vi "LeftButtonUp.vi"(8 "Error in (no error)":errorcluster, 11 "Click?":bool=TRUE) -> (0 "Error out":errorcluster)   [LabVIEW 2013]
uses:
  user32.dll
  Linux VIs/guiLib.so
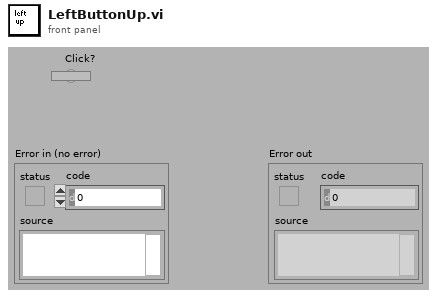
[diagram p1: front panel]
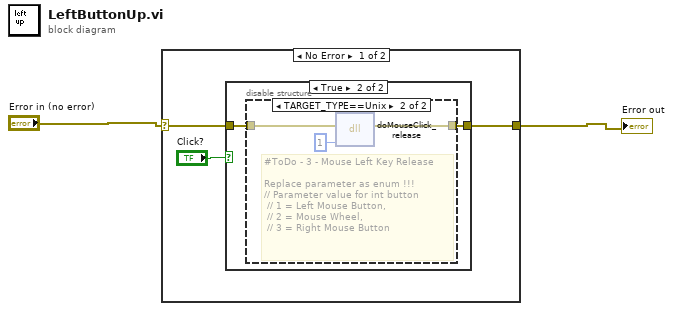
[diagram p0: block diagram]
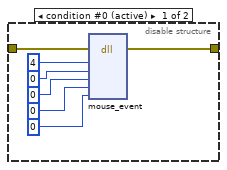
[diagram p3: hidden frame]
diagram:
  n1 = case shown="No Error" "Error in (no error)" {
    selector: "Error in (no error)" -> [w5 w19]
    tunnel: [w4 w19] -> w2
    frame No Error {
      n2 = case shown="True" "Click?" {
        tunnel: w5 -> [w6 w8]
        tunnel: [w6 w7] -> w4
        frame False {
        }
        frame True {
          n3 = disable-structure shown="TARGET_TYPE==Unix" {
            disable-tunnel: w8 -> [w10 w18]
            disable-tunnel: [w9 w17] -> w7
            frame condition #0 (active) {
              n4 = dll-call lib="user32.dll" fn="mouse_event"(error in=w10, "dwFlags"=u32 4, "dx"=u32 0, "dy"=u32 0, "dwData"=u32 0, "dxExtraInfo"=u32 0) -> (error out=w9:errorcluster)  [unwired: 7 in, 2 out]
            }
            frame condition #1 {
              # "#ToDo - 3 - Mouse Left Key Release\n\nReplace parameter as enum !!!\n// Parameter value for int button\n\t// 1 = Left Mouse Button, \n\t// 2 = Mouse Wheel,\n\t// 3 = Right Mouse Button"
              n5 = dll-call lib="home/lvadmin/inmathed_linux_GUI/inmathed_linux_GUI/LabVIEWTestSystems/LV GUI ToolKit/LV GUI 2013/LabVIEW GUI Automation Toolkit/Utility/Linux VIs/guiLib.so" fn="doMouseClick_release"(error in=w18, "Button"=1) -> (error out=w17:errorcluster)  [unwired: 4 in, 1 out]
            }
          }
        }
      }
    }
    frame Error {
    }
  }
  "Error out" <- w2
